vi "Block Tree.vi"   [LabVIEW 2022 SP3]
uses:
  FlexBlocks Support/FlexBlocks Support.lvlib
types:
  T1 = enum32{"Invalid", "Standard", "Closed", "Hidden", "Minimized", "Maximized"}
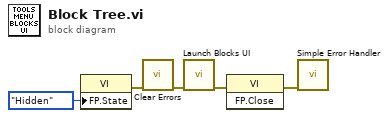
[diagram p0: block diagram]
diagram:
  n1 = property class="VI"("FP.State"=T1."Hidden" ("Front Panel Window:State")) -> (error out=w2:errorcluster)  [unwired: 2 in, 1 out]
  n2 = call <vilib>:"Clear Errors.vi"("error in (no error)"=w2) -> ("error out"=w3:errorcluster)  [unwired: 5 in, 1 out]
  n3 = call "Launch Blocks UI.vi"("error in (no error)"=w3) -> ("error out"=w5:errorcluster)  [unwired: 10 in]
  n4 = invoke class="VI" method="FP.Close"(error in=w5) -> (error out=w4:errorcluster)  [unwired: 2 in, 2 out]
  n5 = call <vilib>:"Simple Error Handler.vi"("error in (no error)"=w4) -> ()  [unwired: 4 in, 5 out]
